vi "Check Shield Time.vi"(8 "error in (no error)":errorcluster, 11 "Shield in":refnum<class "Shield.lvclass">) -> (0 "error out":errorcluster, 3 "Shield out":refnum<class "Shield.lvclass">)   [LabVIEW 2021, in "Shield.lvclass"]
uses:
  Shield.lvclass
  C:/Users/poche/Programs/LabVIEW/imposible snake/GameEl_class/GameEl.lvclass
  Shield.lvclass/Shield.ctl
  GameEl_class/GameEl.lvclass/GameEl.ctl
  GameEl_class/GameEl.lvclass
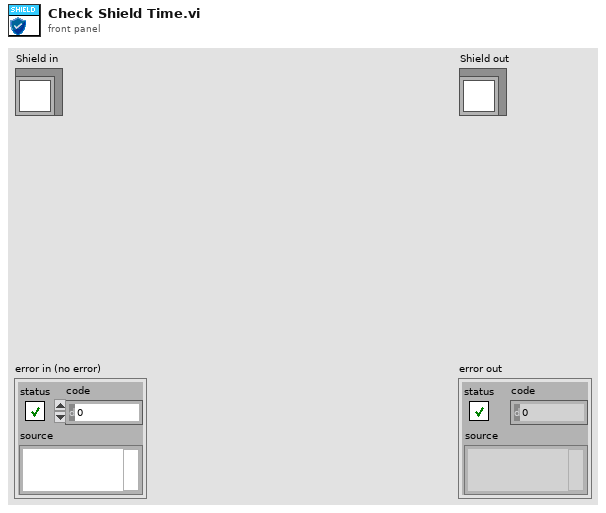
[diagram p1: front panel]
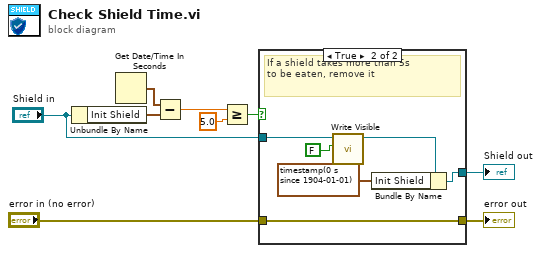
[diagram p0: block diagram]
diagram:
  n1 = Unbundle By Name("Shield in") -> ("Init Shield"=w8:timestamp)
  n2 = Get Date/Time In Seconds() -> (seconds since 1Jan1904=w9:timestamp)
  n3 = Subtract(x=w9, y=w8) -> (x-y=w7:dbl)
  n4 = Greater Or Equal?(x=w7, y=5.0) -> (x >= y?=w1:bool)
  n5 = case shown="True" w1 {
    tunnel: "Shield in" -> [w11 w17]
    tunnel: [w11 w16] -> w4
    tunnel: "error in (no error)" -> [w10 w14]
    tunnel: [w10 w14] -> w2
    frame False {
    }
    frame True {
      # "If a shield takes more than 5s\nto be eaten, remove it"
      n6 = call "Write Visible.vi"("Visible"=FALSE, "GameEl in"=w17) -> ("GameEl out"=w13:refnum<class "Shield.lvclass">)  [unwired: 8 in, 1 out]
      n7 = Bundle By Name(cluster=w13, "Init Shield"=timestamp(0 s since 1904-01-01)) -> (w16:refnum<class "Shield.lvclass">)
    }
  }
  "error out" <- w2
  "Shield out" <- w4
